vi "get fpga resource refnum.vi"(0 "bitfile ref in":refnum<k20>, 5 "channel":refnum<class "TBM channel.lvclass">, 11 "error in (no error)":errorcluster) -> (4 "control ref out":refnum<k20>, 6 "fpga res type":T1, 15 "error out":errorcluster)   [LabVIEW 2015, in "io runtime.lvclass"]
uses:
  io runtime.lvclass
  <vilib>/NI/Tag Bus Module Framework/channel/TBM channel.lvclass
  configuration/fpga resource supported data types.ctl
  configuration/Fxp Channel/Fxp Channel.lvclass
  <vilib>/NI/Tag Bus/tag/tag descriptor.lvclass/tag descriptor.ctl
  configuration/Fxp Channel/Fxp Channel.lvclass/Fxp Channel.ctl
  FXP I_20_5.ctl
  FXP I_24_5.ctl
  FXP I_24_10.ctl
  <vilib>/NI/LVFPGA Adv Session Resources/OpenByNameSubVI.vi
  <vilib>/NI/Tag Bus/tag/read tag name.vi
  configuration/Fxp Channel/Read FXP type.vi
  <vilib>/NI/Tag Bus/tag/read data type.vi
  <vilib>/rvi/interface/common/dynamic/niFpgaEscapeDelimiterAndNull.vi
  <vilib>/Utility/error.llb/Error Cluster From Error Code.vi
  <vilib>/NI/LVFPGA Adv Session Resources/OpenByName.xnode
  <vilib>/NI/LVFPGA Adv Session Resources/LVFPGAAdvSessionResources.lvlib
  configuration/io configuration.lvclass
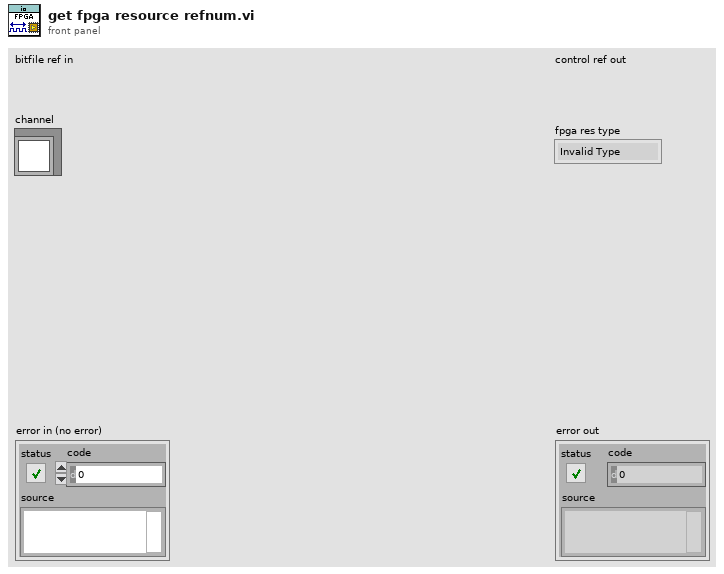
[diagram p1: front panel]
types:
  T1 = typedef "io configuration.lvclass/fpga resource supported data types.ctl" = enum16{"Invalid Type", "Single", "I64", "I32", "I16", "I8", "U64", "U32", "U16", "U8", "Boolean", "I,20,5", "I,24,5", "I,24,10"}
  T2 = cluster{"Name":string, "Depth":u32, "Write? (Deprecated:Use Implementation)":bool, "Physical Channel":u32, "Base Address":u32, "Data Width":u32, "Data Type":enum32{"Boolean", "I8", "I16", "I32", "I64", "U8", "U16", "U32", "U64", "FXP", "CustomControl", "SGL"}, "FXP Properties":variant, "Write Window Address":u32, "Implementation":enum16{"niFpgaTargetToHost", "niFpgaHostToTarget", "niFpgaPeerToPeerWriter", "niFpgaPeerToPeerReader", "niCoreTargetToHost", "niCoreHostToTarget"}, "Control Set":u32}[]
  T3 = cluster{"Name":string, "type":variant, "indicator?":bool}[]
  T4 = typedef "LVFixedPointRepBitsTypeDef.ctl" = cluster{"Signed":bool, "Word Length":u32, "Integer Word Length":i32}
  T5 = typedef "io runtime.lvclass/FXP I_20_5.ctl" = refnum<k20>
  T6 = typedef "io runtime.lvclass/FXP I_24_5.ctl" = refnum<k20>
  T7 = typedef "io runtime.lvclass/FXP I_24_10.ctl" = refnum<k20>
  T8 = typedef "tag bus.lvlib/tag descriptor.lvclass/Data Type.ctl" = enum16{"Double", "Single", "I64", "I32", "I16", "I8", "U64", "U32", "U16", "U8", "Boolean", "String", "Array of Double", "Array of Single", "Array of I64", "Array of I32", "Array of I16", "Array of I8", "Array of U64", "Array of U32", "Array of U16", "Array of U8", "Array of Boolean", "Array of String"}
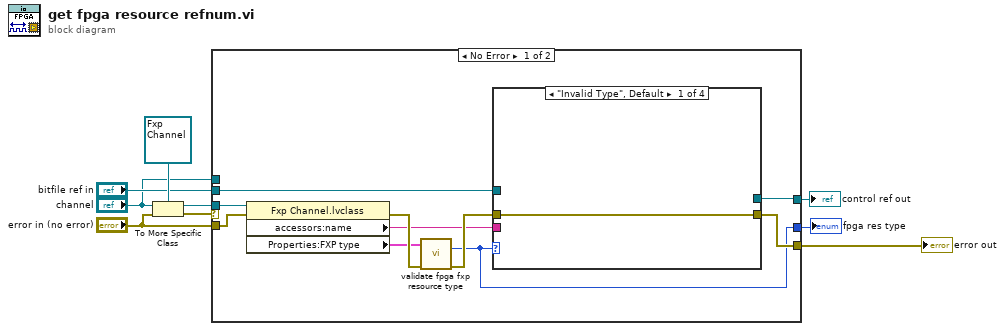
[diagram p0: block diagram]
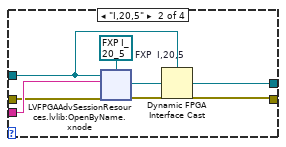
[diagram p2: hidden frame]
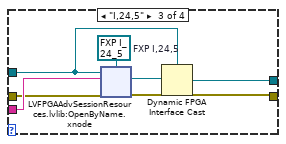
[diagram p3: hidden frame]
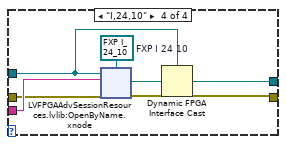
[diagram p4: hidden frame]
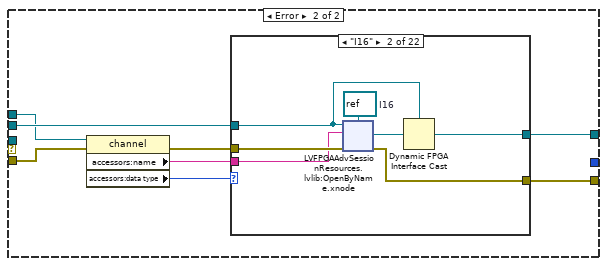
[diagram p5: hidden frame]
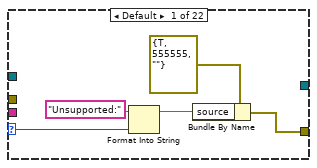
[diagram p6: hidden frame]
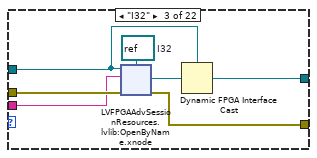
[diagram p7: hidden frame]
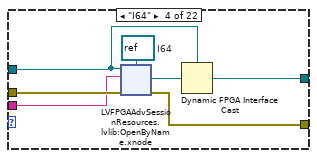
[diagram p8: hidden frame]
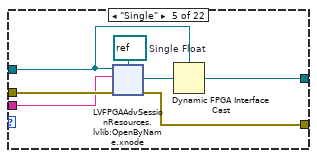
[diagram p9: hidden frame]
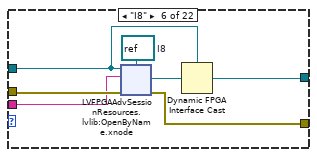
[diagram p10: hidden frame]
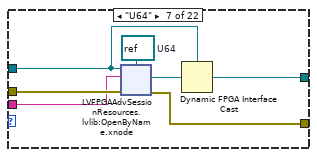
[diagram p11: hidden frame]
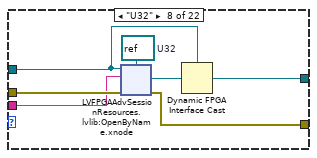
[diagram p12: hidden frame]
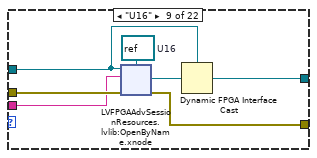
[diagram p13: hidden frame]
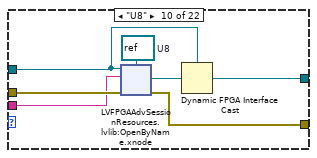
[diagram p14: hidden frame]
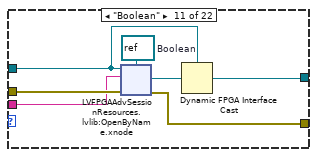
[diagram p15: hidden frame]
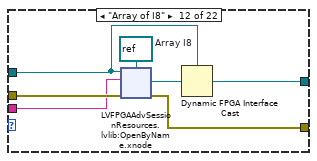
[diagram p16: hidden frame]
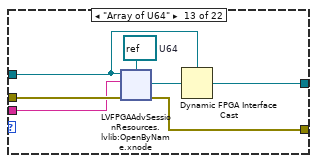
[diagram p17: hidden frame]
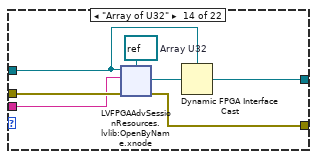
[diagram p18: hidden frame]
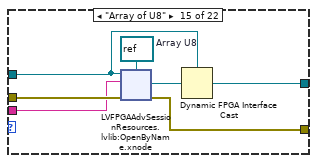
[diagram p19: hidden frame]
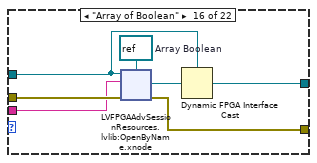
[diagram p20: hidden frame]
diagram:
  n1 = To More Specific Class(target class=refnum<class "Fxp Channel.lvclass"> refnum ("Fxp Channel.lvclass"), reference="channel", error in="error in (no error)") -> (specific class reference=w7:refnum<class "Fxp Channel.lvclass">, error out=w8:errorcluster)
  n2 = case shown="No Error" w8 {
    tunnel: w7 -> [w17 _]
    tunnel: "bitfile ref in" -> [w16 w83]
    tunnel: [w13 w84] -> w1
    tunnel: [w15 w88] -> w4
    tunnel: [w11 _] -> w5
    tunnel: "channel" -> [_ w82]
    tunnel: "error in (no error)" -> [w10 w81]
    frame No Error {
      n3 = property class="Fxp Channel.lvclass"(reference=w17, error in=w10) -> (error out=w19:errorcluster, "accessors:name"=w14:string, "Properties:FXP type"=w12:T4)  [unwired: 1 out]
      n4 = call "validate fpga fxp resource type.vi"("FXP Representation"=w12, "error in (no error)"=w19) -> ("fpga res type"=w11:T1, "error out"=w18:errorcluster)  [unwired: 11 in, 1 out]
      n5 = case shown="\"Invalid Type\", Default" w11 {
        tunnel: w16 -> [_ w22 w47 w66]
        tunnel: [_ w26 w46 w65] -> w15
        tunnel: w14 -> [_ w25 w45 w64]
        tunnel: w18 -> [w20 w24 w44 w63]
        tunnel: [w20 w23 w43 w62] -> w13
        frame "Invalid Type", Default {
        }
        frame "I,20,5" {
          w21 = T5 refnum  # FXP  I,20,5
          n6 = xnode "LVFPGAAdvSessionResources.lvlib:OpenByName.xnode"("FPGA VI Reference in"=w22, "Resource name in"=w25, "Single resource reference type in"=w21, "Error in"=w24) -> ("Single resource reference out"=w27:T5, "Error out"=w23:errorcluster)  [unwired: 1 out]
          n7 = Dynamic FPGA Interface Cast(Session In=w22, Type=w27) -> (Session Out=w26:refnum<k20>)
        }
        frame "I,24,5" {
          w41 = T6 refnum  # FXP I,24,5
          n8 = xnode "LVFPGAAdvSessionResources.lvlib:OpenByName.xnode"("FPGA VI Reference in"=w47, "Resource name in"=w45, "Single resource reference type in"=w41, "Error in"=w44) -> ("Single resource reference out"=w42:T6, "Error out"=w43:errorcluster)  [unwired: 1 out]
          n9 = Dynamic FPGA Interface Cast(Session In=w47, Type=w42) -> (Session Out=w46:refnum<k20>)
        }
        frame "I,24,10" {
          w61 = T7 refnum  # FXP I 24 10
          n10 = xnode "LVFPGAAdvSessionResources.lvlib:OpenByName.xnode"("FPGA VI Reference in"=w66, "Resource name in"=w64, "Single resource reference type in"=w61, "Error in"=w63) -> ("Single resource reference out"=w67:T7, "Error out"=w62:errorcluster)  [unwired: 1 out]
          n11 = Dynamic FPGA Interface Cast(Session In=w66, Type=w67) -> (Session Out=w65:refnum<k20>)
        }
      }
    }
    frame Error {
      n12 = property class="channel"(reference=w82, error in=w81) -> (error out=w87:errorcluster, "accessors:name"=w85:string, "accessors:data type"=w86:T8)  [unwired: 1 out]
      n13 = case shown="\"I16\"" w86 {
        selector: w86 -> [w91 _ _ _ _ _ _ _ _ _ _ _ _ _ _ _ _ _ _ _ _ _]
        tunnel: w87 -> [_ w100 w120 w140 w160 w180 w200 w220 w240 w260 w280 w300 w320 w340 w360 w380 w400 w420 w440 w460 w480 w500]
        tunnel: [w93 w99 w119 w139 w159 w179 w199 w219 w239 w259 w279 w299 w319 w339 w359 w379 w399 w414 w439 w459 w479 w499] -> w84
        tunnel: w83 -> [_ w97 w117 w137 w157 w177 w197 w217 w237 w257 w277 w297 w317 w337 w357 w377 w396 w417 w436 w456 w476 w496]
        tunnel: w85 -> [_ w98 w118 w138 w158 w178 w198 w218 w238 w258 w278 w298 w318 w338 w358 w378 w398 w419 w438 w458 w478 w498]
        tunnel: [_ w96 w116 w136 w156 w176 w196 w216 w236 w256 w276 w296 w316 w336 w356 w376 w395 w416 w435 w455 w475 w495] -> w88
        frame Default {
          n14 = Format Into String(initial string="Unsupported:" ("source"), w91) -> (resulting string=w89:string)  [unwired: 2 in, 1 out]
          n15 = Bundle By Name(cluster=errorcluster {"status"=TRUE, "code"=555555, "source"=""} ("Error out"), "source"=w89) -> (w93:errorcluster)
        }
        frame "I16" {
          w95 = refnum<k20> refnum  # I16
          n16 = xnode "LVFPGAAdvSessionResources.lvlib:OpenByName.xnode"("FPGA VI Reference in"=w97, "Resource name in"=w98, "Single resource reference type in"=w95, "Error in"=w100) -> ("Single resource reference out"=w94:refnum<k20>, "Error out"=w99:errorcluster)  [unwired: 1 out]
          n17 = Dynamic FPGA Interface Cast(Session In=w97, Type=w94) -> (Session Out=w96:refnum<k20>)
        }
        frame "I32" {
          w115 = refnum<k20> refnum  # I32
          n18 = xnode "LVFPGAAdvSessionResources.lvlib:OpenByName.xnode"("FPGA VI Reference in"=w117, "Resource name in"=w118, "Single resource reference type in"=w115, "Error in"=w120) -> ("Single resource reference out"=w114:refnum<k20>, "Error out"=w119:errorcluster)  [unwired: 1 out]
          n19 = Dynamic FPGA Interface Cast(Session In=w117, Type=w114) -> (Session Out=w116:refnum<k20>)
        }
        frame "I64" {
          w135 = refnum<k20> refnum  # I64
          n20 = xnode "LVFPGAAdvSessionResources.lvlib:OpenByName.xnode"("FPGA VI Reference in"=w137, "Resource name in"=w138, "Single resource reference type in"=w135, "Error in"=w140) -> ("Single resource reference out"=w134:refnum<k20>, "Error out"=w139:errorcluster)  [unwired: 1 out]
          n21 = Dynamic FPGA Interface Cast(Session In=w137, Type=w134) -> (Session Out=w136:refnum<k20>)
        }
        frame "Single" {
          w155 = refnum<k20> refnum  # Single Float
          n22 = xnode "LVFPGAAdvSessionResources.lvlib:OpenByName.xnode"("FPGA VI Reference in"=w157, "Resource name in"=w158, "Single resource reference type in"=w155, "Error in"=w160) -> ("Single resource reference out"=w154:refnum<k20>, "Error out"=w159:errorcluster)  [unwired: 1 out]
          n23 = Dynamic FPGA Interface Cast(Session In=w157, Type=w154) -> (Session Out=w156:refnum<k20>)
        }
        frame "I8" {
          w175 = refnum<k20> refnum  # I8
          n24 = xnode "LVFPGAAdvSessionResources.lvlib:OpenByName.xnode"("FPGA VI Reference in"=w177, "Resource name in"=w178, "Single resource reference type in"=w175, "Error in"=w180) -> ("Single resource reference out"=w174:refnum<k20>, "Error out"=w179:errorcluster)  [unwired: 1 out]
          n25 = Dynamic FPGA Interface Cast(Session In=w177, Type=w174) -> (Session Out=w176:refnum<k20>)
        }
        frame "U64" {
          w195 = refnum<k20> refnum  # U64
          n26 = xnode "LVFPGAAdvSessionResources.lvlib:OpenByName.xnode"("FPGA VI Reference in"=w197, "Resource name in"=w198, "Single resource reference type in"=w195, "Error in"=w200) -> ("Single resource reference out"=w194:refnum<k20>, "Error out"=w199:errorcluster)  [unwired: 1 out]
          n27 = Dynamic FPGA Interface Cast(Session In=w197, Type=w194) -> (Session Out=w196:refnum<k20>)
        }
        frame "U32" {
          w215 = refnum<k20> refnum  # U32
          n28 = xnode "LVFPGAAdvSessionResources.lvlib:OpenByName.xnode"("FPGA VI Reference in"=w217, "Resource name in"=w218, "Single resource reference type in"=w215, "Error in"=w220) -> ("Single resource reference out"=w214:refnum<k20>, "Error out"=w219:errorcluster)  [unwired: 1 out]
          n29 = Dynamic FPGA Interface Cast(Session In=w217, Type=w214) -> (Session Out=w216:refnum<k20>)
        }
        frame "U16" {
          w235 = refnum<k20> refnum  # U16
          n30 = xnode "LVFPGAAdvSessionResources.lvlib:OpenByName.xnode"("FPGA VI Reference in"=w237, "Resource name in"=w238, "Single resource reference type in"=w235, "Error in"=w240) -> ("Single resource reference out"=w234:refnum<k20>, "Error out"=w239:errorcluster)  [unwired: 1 out]
          n31 = Dynamic FPGA Interface Cast(Session In=w237, Type=w234) -> (Session Out=w236:refnum<k20>)
        }
        frame "U8" {
          w255 = refnum<k20> refnum  # U8
          n32 = xnode "LVFPGAAdvSessionResources.lvlib:OpenByName.xnode"("FPGA VI Reference in"=w257, "Resource name in"=w258, "Single resource reference type in"=w255, "Error in"=w260) -> ("Single resource reference out"=w254:refnum<k20>, "Error out"=w259:errorcluster)  [unwired: 1 out]
          n33 = Dynamic FPGA Interface Cast(Session In=w257, Type=w254) -> (Session Out=w256:refnum<k20>)
        }
        frame "Boolean" {
          w275 = refnum<k20> refnum  # Boolean
          n34 = xnode "LVFPGAAdvSessionResources.lvlib:OpenByName.xnode"("FPGA VI Reference in"=w277, "Resource name in"=w278, "Single resource reference type in"=w275, "Error in"=w280) -> ("Single resource reference out"=w274:refnum<k20>, "Error out"=w279:errorcluster)  [unwired: 1 out]
          n35 = Dynamic FPGA Interface Cast(Session In=w277, Type=w274) -> (Session Out=w276:refnum<k20>)
        }
        frame "Array of I8" {
          w294 = refnum<k20> refnum  # Array I8
          n36 = xnode "LVFPGAAdvSessionResources.lvlib:OpenByName.xnode"("FPGA VI Reference in"=w297, "Resource name in"=w298, "Single resource reference type in"=w294, "Error in"=w300) -> ("Single resource reference out"=w295:refnum<k20>, "Error out"=w299:errorcluster)  [unwired: 1 out]
          n37 = Dynamic FPGA Interface Cast(Session In=w297, Type=w295) -> (Session Out=w296:refnum<k20>)
        }
        frame "Array of U64" {
          w314 = refnum<k20> refnum  # U64
          n38 = xnode "LVFPGAAdvSessionResources.lvlib:OpenByName.xnode"("FPGA VI Reference in"=w317, "Resource name in"=w318, "Single resource reference type in"=w314, "Error in"=w320) -> ("Single resource reference out"=w315:refnum<k20>, "Error out"=w319:errorcluster)  [unwired: 1 out]
          n39 = Dynamic FPGA Interface Cast(Session In=w317, Type=w315) -> (Session Out=w316:refnum<k20>)
        }
        frame "Array of U32" {
          w334 = refnum<k20> refnum  # Array U32
          n40 = xnode "LVFPGAAdvSessionResources.lvlib:OpenByName.xnode"("FPGA VI Reference in"=w337, "Resource name in"=w338, "Single resource reference type in"=w334, "Error in"=w340) -> ("Single resource reference out"=w335:refnum<k20>, "Error out"=w339:errorcluster)  [unwired: 1 out]
          n41 = Dynamic FPGA Interface Cast(Session In=w337, Type=w335) -> (Session Out=w336:refnum<k20>)
        }
        frame "Array of U8" {
          w354 = refnum<k20> refnum  # Array U8
          n42 = xnode "LVFPGAAdvSessionResources.lvlib:OpenByName.xnode"("FPGA VI Reference in"=w357, "Resource name in"=w358, "Single resource reference type in"=w354, "Error in"=w360) -> ("Single resource reference out"=w355:refnum<k20>, "Error out"=w359:errorcluster)  [unwired: 1 out]
          n43 = Dynamic FPGA Interface Cast(Session In=w357, Type=w355) -> (Session Out=w356:refnum<k20>)
        }
        frame "Array of Boolean" {
          w374 = refnum<k20> refnum  # Array Boolean
          n44 = xnode "LVFPGAAdvSessionResources.lvlib:OpenByName.xnode"("FPGA VI Reference in"=w377, "Resource name in"=w378, "Single resource reference type in"=w374, "Error in"=w380) -> ("Single resource reference out"=w375:refnum<k20>, "Error out"=w379:errorcluster)  [unwired: 1 out]
          n45 = Dynamic FPGA Interface Cast(Session In=w377, Type=w375) -> (Session Out=w376:refnum<k20>)
        }
        frame "Array of Single" {
          w394 = refnum<k20> refnum  # Array Single
          n46 = xnode "LVFPGAAdvSessionResources.lvlib:OpenByName.xnode"("FPGA VI Reference in"=w396, "Resource name in"=w398, "Single resource reference type in"=w394, "Error in"=w400) -> ("Single resource reference out"=w397:refnum<k20>, "Error out"=w399:errorcluster)  [unwired: 1 out]
          n47 = Dynamic FPGA Interface Cast(Session In=w396, Type=w397) -> (Session Out=w395:refnum<k20>)
        }
        frame "Array of Double" {
          w415 = refnum<k20> refnum  # FXP
          n48 = xnode "LVFPGAAdvSessionResources.lvlib:OpenByName.xnode"("FPGA VI Reference in"=w417, "Resource name in"=w419, "Single resource reference type in"=w415, "Error in"=w420) -> ("Single resource reference out"=w418:refnum<k20>, "Error out"=w414:errorcluster)  [unwired: 1 out]
          n49 = Dynamic FPGA Interface Cast(Session In=w417, Type=w418) -> (Session Out=w416:refnum<k20>)
        }
        frame "Array of I64" {
          w434 = refnum<k20> refnum  # Array I64
          n50 = xnode "LVFPGAAdvSessionResources.lvlib:OpenByName.xnode"("FPGA VI Reference in"=w436, "Resource name in"=w438, "Single resource reference type in"=w434, "Error in"=w440) -> ("Single resource reference out"=w437:refnum<k20>, "Error out"=w439:errorcluster)  [unwired: 1 out]
          n51 = Dynamic FPGA Interface Cast(Session In=w436, Type=w437) -> (Session Out=w435:refnum<k20>)
        }
        frame "Array of I32" {
          w454 = refnum<k20> refnum  # Array I32
          n52 = xnode "LVFPGAAdvSessionResources.lvlib:OpenByName.xnode"("FPGA VI Reference in"=w456, "Resource name in"=w458, "Single resource reference type in"=w454, "Error in"=w460) -> ("Single resource reference out"=w457:refnum<k20>, "Error out"=w459:errorcluster)  [unwired: 1 out]
          n53 = Dynamic FPGA Interface Cast(Session In=w456, Type=w457) -> (Session Out=w455:refnum<k20>)
        }
        frame "Array of I16" {
          w474 = refnum<k20> refnum  # Array I16
          n54 = xnode "LVFPGAAdvSessionResources.lvlib:OpenByName.xnode"("FPGA VI Reference in"=w476, "Resource name in"=w478, "Single resource reference type in"=w474, "Error in"=w480) -> ("Single resource reference out"=w477:refnum<k20>, "Error out"=w479:errorcluster)  [unwired: 1 out]
          n55 = Dynamic FPGA Interface Cast(Session In=w476, Type=w477) -> (Session Out=w475:refnum<k20>)
        }
        frame "Array of U16" {
          w494 = refnum<k20> refnum  # Array U16
          n56 = xnode "LVFPGAAdvSessionResources.lvlib:OpenByName.xnode"("FPGA VI Reference in"=w496, "Resource name in"=w498, "Single resource reference type in"=w494, "Error in"=w500) -> ("Single resource reference out"=w497:refnum<k20>, "Error out"=w499:errorcluster)  [unwired: 1 out]
          n57 = Dynamic FPGA Interface Cast(Session In=w496, Type=w497) -> (Session Out=w495:refnum<k20>)
        }
      }
    }
  }
  "error out" <- w1
  "control ref out" <- w4
  "fpga res type" <- w5
